vi "PatManage.vi"() -> ()   [LabVIEW 2012]
panel:
  in  "print":bool
  out "簇":T1
  in  "delete":bool
  in  "add":bool
  in  "ShowAll":bool
  in  "find":u16(ring) items=["请选择查询方式", "编号查询", "姓名查询", "性别查询", "年龄查询", "病区/床号查询", "治疗模式查询", "治疗次数查询", "治疗时长查询", "治疗日期查询"]
  out "查找结果":string
  in  "病历显示":string[][](table)
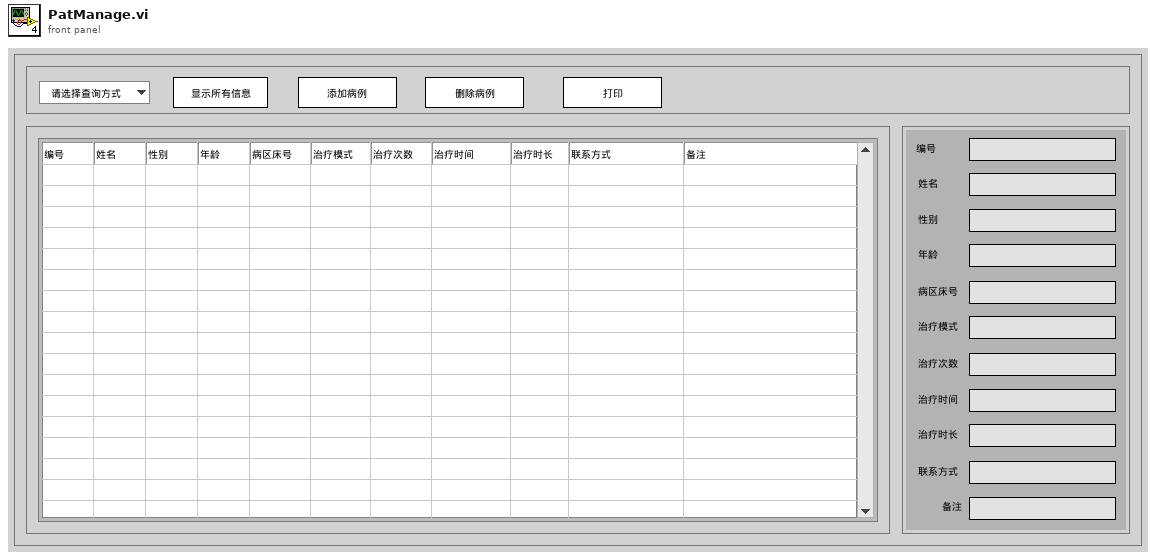
[diagram p1: front panel]
types:
  T1 = cluster{"编号":string, "姓名":string, "性别":string, "年龄":string, "病区床号":string, "治疗模式":string, "治疗次数":string, "治疗时间":string, "治疗时长":string, "联系方式":string, "备注":string}
  T2 = typedef "LVRowAndColumnTypeDef.ctl" = cluster{"Row":i32, "Column":i32}
  T3 = cluster{string, string, string, string, string, string, string, string, string, string, string}
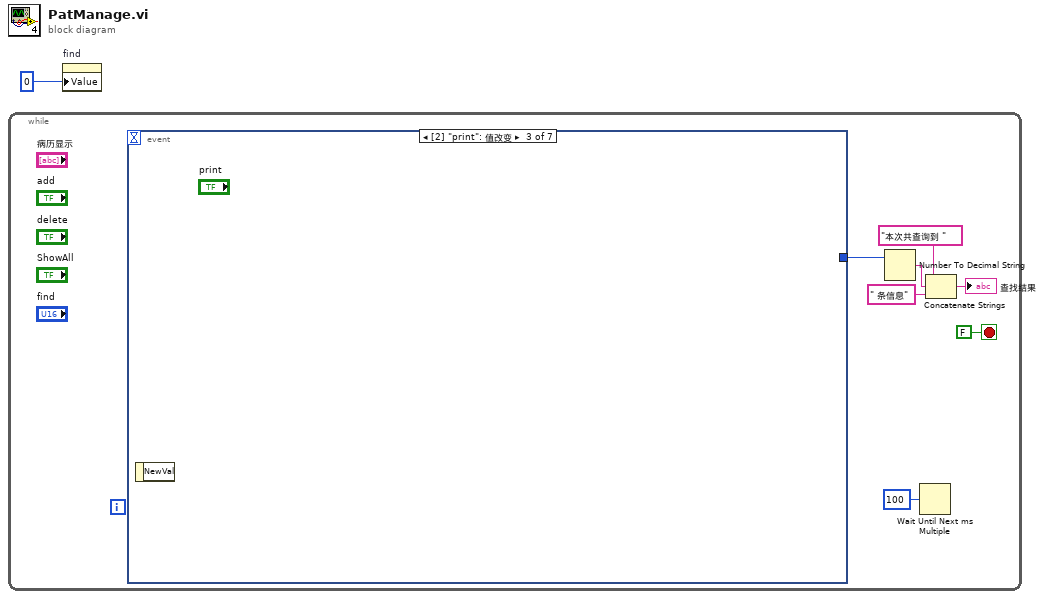
[diagram p0: block diagram]
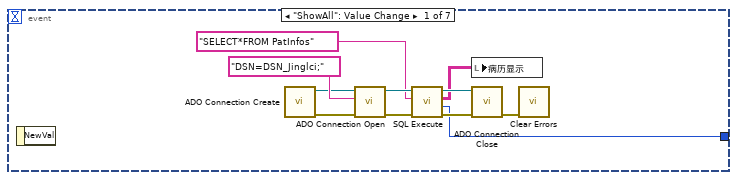
[diagram p2: hidden frame]
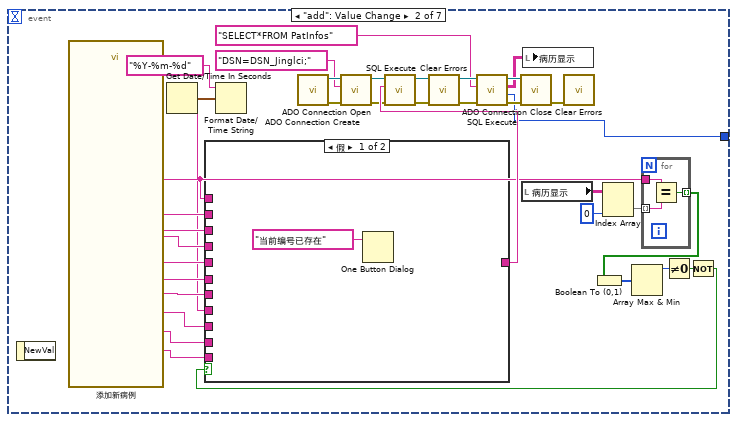
[diagram p3: hidden frame]
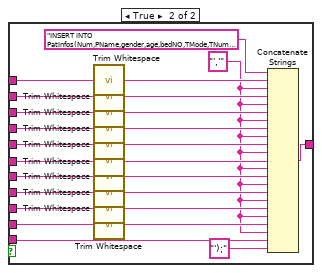
[diagram p4: hidden frame]
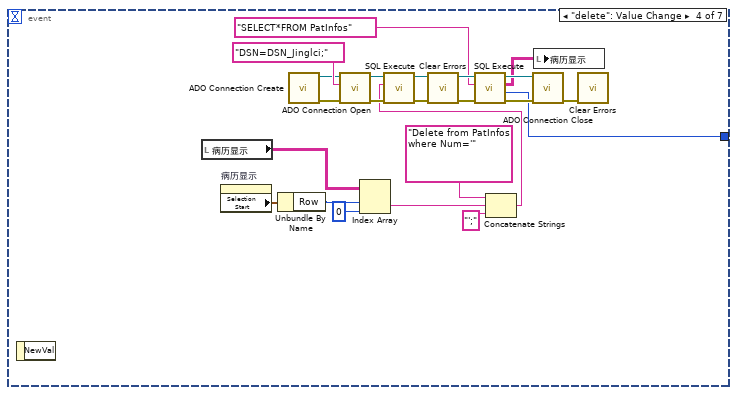
[diagram p5: hidden frame]
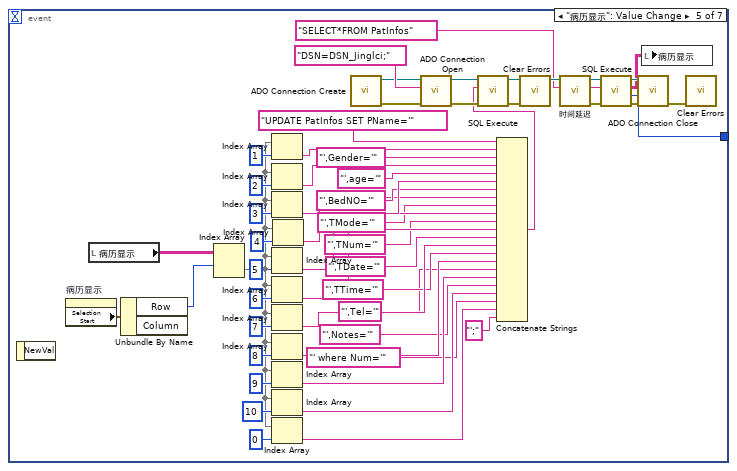
[diagram p6: hidden frame]
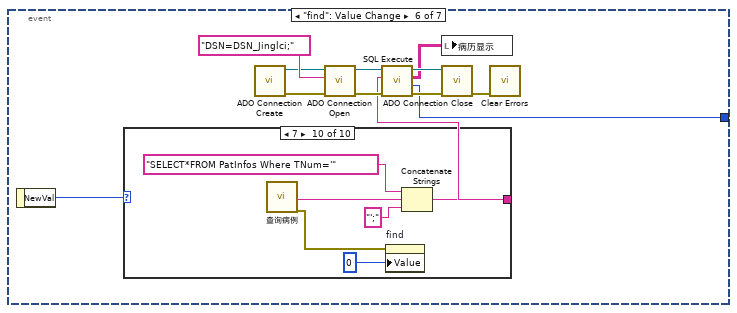
[diagram p7: hidden frame]
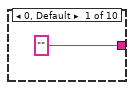
[diagram p8: hidden frame]
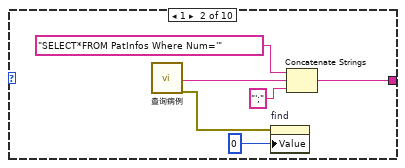
[diagram p9: hidden frame]
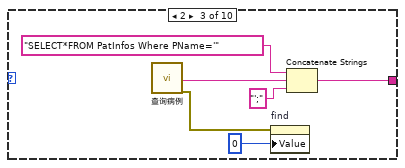
[diagram p10: hidden frame]
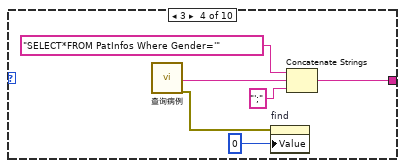
[diagram p11: hidden frame]
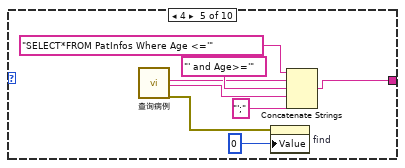
[diagram p12: hidden frame]
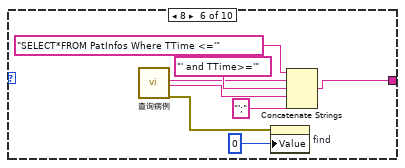
[diagram p13: hidden frame]
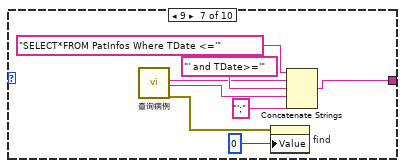
[diagram p14: hidden frame]
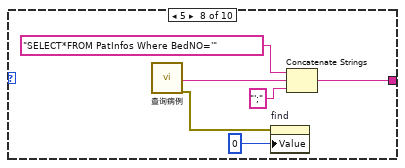
[diagram p15: hidden frame]
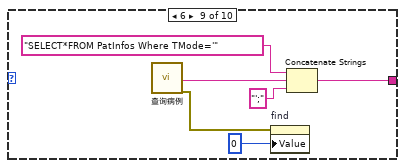
[diagram p16: hidden frame]
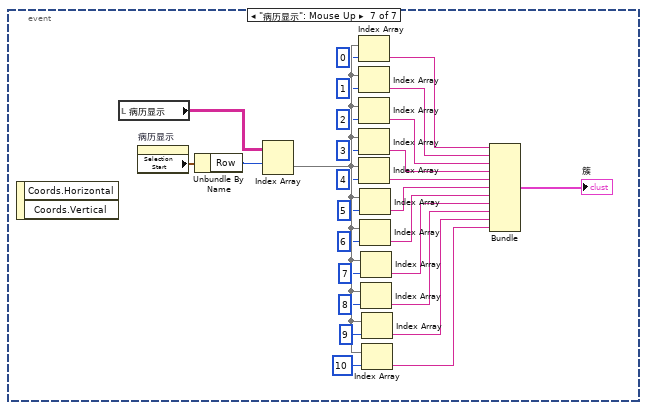
[diagram p17: hidden frame]
diagram:
  n1 = while {
    stop <- FALSE stop-if-true
    n2 = event shown="[2] \"print\": 值改变" {
      selector: _ -> [_ _ _ _ _ _ _]
      dyn-events: _ -> [_ _ _ _ _ _ _]
      timeout: _ -> [_ _ _ _ _ _ _]
      tunnel: [w9 w37 _ w88 w148 w160 _] -> w2
      event "ShowAll": Value Change {
        n3 = event-data() -> ()  [unwired: 1 in, 1 out]
        n4 = call "ADO Connection Create.vi"() -> ("error out"=w14:errorcluster, "ADODB._Connection Out"=w13:refnum<k7>)  [unwired: 10 in]
        n5 = call "ADO Connection Open.vi"("error in (no error)"=w14, "ConnectionString"="DSN=DSN_Jinglci;" ("Command Text"), "ADODB._Connection In"=w13) -> ("error out"=w19:errorcluster, "ADODB._Connection Out"=w18:refnum<k7>)  [unwired: 7 in]
        n6 = call "SQL Execute.vi"("error in (no error)"=w19, "Command Text"="SELECT*FROM PatInfos", "ADODB._Connection In"=w18) -> ("error out"=w15:errorcluster, "Rows Fetched"=w9:i32, "Data"=w10:string[][], "ADODB._Connection Out"=w17:refnum<k7>)  [unwired: 5 in]
        n7 = local write "病历显示"(w10) -> ()
        n8 = call "ADO Connection Close.vi"("error in (no error)"=w15, "ADODB._Connection In"=w17) -> ("error out"=w11:errorcluster)  [unwired: 8 in, 1 out]
        n9 = call <vilib>:"Clear Errors.vi"("error in (no error)"=w11) -> ()  [unwired: 6 in, 1 out]
      }
      event "add": Value Change {
        n10 = event-data() -> ()  [unwired: 1 in, 1 out]
        n11 = call "添加新病例"() -> ("备注"=w25:string, "联系方式"=w26:string, "治疗时长"=w22:string, "治疗次数"=w50:string, "治疗模式"=w51:string, "病区/床号"=w52:string, "年龄"=w53:string, "性别"=w54:string, "姓名"=w55:string, "编号"=w32:string)  [unwired: 8 in, 2 out]
        n12 = Get Date/Time In Seconds() -> (seconds since 1Jan1904=w24:timestamp)
        n13 = Format Date/Time String(time format string (%c)="%Y-%m-%d" ("时间格式字符串(%c)"), seconds (now)=w24) -> (date/time string=w21:string)  [unwired: 1 in]
        n14 = call "ADO Connection Create.vi"() -> ("error out"=w45:errorcluster, "ADODB._Connection Out"=w49:refnum<k7>)  [unwired: 10 in]
        n15 = call "ADO Connection Open.vi"("error in (no error)"=w45, "ConnectionString"="DSN=DSN_Jinglci;" ("Command Text"), "ADODB._Connection In"=w49) -> ("error out"=w44:errorcluster, "ADODB._Connection Out"=w47:refnum<k7>)  [unwired: 7 in]
        n16 = local read "病历显示"() -> (w34:string[][])
        n17 = Index Array(array=w34, index (col)=0 ("禁用的索引 (列)")) -> (element=w31:string[])  [unwired: 1 in]
        n18 = for {
          tunnel: w32 -> [w58]
          tunnel: w31 -> [w57] mode=indexing
          tunnel: [w56] -> w28 mode=indexing
          n19 = Equal?(x=w58, y=w57) -> (x = y?=w56:bool)
        }
        n20 = Boolean To (0,1)(Boolean=w28) -> (0, 1=w29:i16[])
        n21 = Array Max & Min(array=w29) -> (max value=w30:i16)  [unwired: 3 out]
        n22 = Not Equal To 0?(x=w30) -> (x != 0?=w27:bool)
        n23 = Not(x=w27) -> (.not. x?=w20:bool)
        n24 = case shown="假" w20 {
          tunnel: w32 -> [_ w84]
          tunnel: w55 -> [_ w83]
          tunnel: w54 -> [_ w82]
          tunnel: w53 -> [_ w81]
          tunnel: w52 -> [_ w80]
          tunnel: w51 -> [_ w79]
          tunnel: w50 -> [_ w78]
          tunnel: w21 -> [_ w77]
          tunnel: [_ w76] -> w46
          tunnel: w26 -> [_ w66]
          tunnel: w25 -> [_ w63]
          tunnel: w22 -> [_ w61]
          frame False {
            n25 = One Button Dialog(message="当前编号已存在" ("消息")) -> ()  [unwired: 1 in, 1 out]
          }
          frame True {
            w64 = "','"
            n26 = call <vilib>:"Trim Whitespace.vi"("string"=w84) -> ("trimmed string"=w75:string)  [unwired: 1 in]
            n27 = call <vilib>:"Trim Whitespace.vi"("string"=w83) -> ("trimmed string"=w74:string)  [unwired: 1 in]
            n28 = call <vilib>:"Trim Whitespace.vi"("string"=w82) -> ("trimmed string"=w73:string)  [unwired: 1 in]
            n29 = call <vilib>:"Trim Whitespace.vi"("string"=w81) -> ("trimmed string"=w72:string)  [unwired: 1 in]
            n30 = call <vilib>:"Trim Whitespace.vi"("string"=w80) -> ("trimmed string"=w71:string)  [unwired: 1 in]
            n31 = call <vilib>:"Trim Whitespace.vi"("string"=w79) -> ("trimmed string"=w70:string)  [unwired: 1 in]
            n32 = call <vilib>:"Trim Whitespace.vi"("string"=w78) -> ("trimmed string"=w69:string)  [unwired: 1 in]
            n33 = call <vilib>:"Trim Whitespace.vi"("string"=w77) -> ("trimmed string"=w68:string)  [unwired: 1 in]
            n34 = call <vilib>:"Trim Whitespace.vi"("string"=w61) -> ("trimmed string"=w67:string)  [unwired: 1 in]
            n35 = call <vilib>:"Trim Whitespace.vi"("string"=w66) -> ("trimmed string"=w65:string)  [unwired: 1 in]
            n36 = Concatenate Strings("INSERT INTO PatInfos(Num,PName,gender,age,bedNO,TMode,TNum,TDate,TTime,Tel,notes)VALUES('" ("Command Text"), w75, w64, w74, w64, w73, w64, w72, w64, w71, w64, w70, w64, w69, w64, w68, w64, w67, w64, w65, w64, w63, "');") -> (w76:string)
          }
        }
        n37 = call "SQL Execute.vi"("error in (no error)"=w44, "Command Text"=w46, "ADODB._Connection In"=w47) -> ("error out"=w42:errorcluster, "ADODB._Connection Out"=w41:refnum<k7>)  [unwired: 5 in, 2 out]
        n38 = call <vilib>:"Clear Errors.vi"("error in (no error)"=w42) -> ("error out"=w35:errorcluster)  [unwired: 6 in]
        n39 = call "SQL Execute.vi"("error in (no error)"=w35, "Command Text"="SELECT*FROM PatInfos", "ADODB._Connection In"=w41) -> ("error out"=w39:errorcluster, "Rows Fetched"=w37:i32, "Data"=w38:string[][], "ADODB._Connection Out"=w40:refnum<k7>)  [unwired: 5 in]
        n40 = call "ADO Connection Close.vi"("error in (no error)"=w39, "ADODB._Connection In"=w40) -> ("error out"=w43:errorcluster)  [unwired: 8 in, 1 out]
        n41 = local write "病历显示"(w38) -> ()
        n42 = call <vilib>:"Clear Errors.vi"("error in (no error)"=w43) -> ()  [unwired: 6 in, 1 out]
      }
      event "print": Value Change {
        n43 = event-data() -> ()  [unwired: 1 in, 1 out]
      }
      event "delete": Value Change {
        n44 = event-data() -> ()  [unwired: 1 in, 1 out]
        n45 = local read "病历显示"() -> (w103:string[][])
        n46 = property on="病历显示" class="Tbl (严格)"() -> ("Selection Start"=w106:T2)  [unwired: 2 in, 2 out]
        n47 = Unbundle By Name(w106) -> ("Row"=w104:i32)
        n48 = call "ADO Connection Create.vi"() -> ("error out"=w96:errorcluster, "ADODB._Connection Out"=w97:refnum<k7>)  [unwired: 10 in]
        n49 = call "ADO Connection Open.vi"("error in (no error)"=w96, "ConnectionString"="DSN=DSN_Jinglci;" ("Command Text"), "ADODB._Connection In"=w97) -> ("error out"=w95:errorcluster, "ADODB._Connection Out"=w99:refnum<k7>)  [unwired: 7 in]
        n50 = Index Array(array=w103, index (row)=w104, index (col)=0 ("disabled index (col)")) -> (element=w102:string)
        n51 = Concatenate Strings("Delete from PatInfos where Num='" ("SQL Text"), w102, "';" ("string")) -> (w93:string)
        n52 = call "SQL Execute.vi"("error in (no error)"=w95, "Command Text"=w93, "ADODB._Connection In"=w99) -> ("error out"=w86:errorcluster, "ADODB._Connection Out"=w92:refnum<k7>)  [unwired: 5 in, 2 out]
        n53 = call <vilib>:"Clear Errors.vi"("error in (no error)"=w86) -> ("error out"=w85:errorcluster)  [unwired: 6 in]
        n54 = call "SQL Execute.vi"("error in (no error)"=w85, "Command Text"="SELECT*FROM PatInfos", "ADODB._Connection In"=w92) -> ("error out"=w90:errorcluster, "Rows Fetched"=w88:i32, "Data"=w89:string[][], "ADODB._Connection Out"=w91:refnum<k7>)  [unwired: 5 in]
        n55 = call "ADO Connection Close.vi"("error in (no error)"=w90, "ADODB._Connection In"=w91) -> ("error out"=w94:errorcluster)  [unwired: 8 in, 1 out]
        n56 = local write "病历显示"(w89) -> ()
        n57 = call <vilib>:"Clear Errors.vi"("error in (no error)"=w94) -> ()  [unwired: 6 in, 1 out]
      }
      event "病历显示": Value Change {
        n58 = event-data() -> ()  [unwired: 1 in, 1 out]
        n59 = property on="病历显示" class="Tbl (严格)"() -> ("Selection Start"=w147:T2)  [unwired: 2 in, 2 out]
        n60 = local read "病历显示"() -> (w146:string[][])
        n61 = Unbundle By Name(w147) -> ("Row"=w145:i32)  [unwired: 1 out]
        n62 = Index Array(array=w146, index (row)=w145) -> (element=w112:string[])  [unwired: 1 in]
        n63 = Index Array(array=w112, index=1 ("索引")) -> (element=w126:string)
        n64 = Index Array(array=w112, index=2 ("索引")) -> (element=w140:string)
        n65 = Index Array(array=w112, index=3 ("索引")) -> (element=w137:string)
        n66 = Index Array(array=w112, index=5 ("索引")) -> (element=w132:string)
        n67 = Index Array(array=w112, index=6 ("索引")) -> (element=w130:string)
        n68 = Index Array(array=w112, index=7 ("索引")) -> (element=w124:string)
        n69 = Index Array(array=w112, index=8 ("索引")) -> (element=w121:string)
        n70 = Index Array(array=w112, index=9 ("索引")) -> (element=w119:string)
        n71 = Index Array(array=w112, index=10 ("索引")) -> (element=w113:string)
        n72 = Index Array(array=w112, index=0 ("索引")) -> (element=w111:string)
        n73 = Index Array(array=w112, index=4 ("索引")) -> (element=w134:string)
        n74 = call "ADO Connection Create.vi"() -> ("error out"=w156:errorcluster, "ADODB._Connection Out"=w155:refnum<k7>)  [unwired: 10 in]
        n75 = call "ADO Connection Open.vi"("error in (no error)"=w156, "ConnectionString"="DSN=DSN_Jinglci;" ("Command Text"), "ADODB._Connection In"=w155) -> ("error out"=w159:errorcluster, "ADODB._Connection Out"=w158:refnum<k7>)  [unwired: 7 in]
        n76 = Concatenate Strings("UPDATE PatInfos SET PName='" ("Command Text"), w126, "',Gender='" ("字符串"), w140, "',age='" ("字符串"), w137, "',BedNO='" ("字符串"), w134, "',TMode='" ("字符串"), w132, "',TNum='" ("字符串"), w130, "',TDate='" ("字符串"), w124, "',TTime='" ("字符串"), w121, "',Tel='" ("字符串"), w119, "',Notes='" ("字符串"), w113, "' where Num='" ("字符串"), w111, "';" ("字符串")) -> (w118:string)
        n77 = call "SQL Execute.vi"("error in (no error)"=w159, "Command Text"=w118, "ADODB._Connection In"=w158) -> ("error out"=w117:errorcluster, "ADODB._Connection Out"=w153:refnum<k7>)  [unwired: 5 in, 2 out]
        n78 = call <vilib>:"Clear Errors.vi"("error in (no error)"=w117) -> ()  [unwired: 6 in, 1 out]
        n79 = call "时间延迟"() -> ("error out"=w116:errorcluster)  [unwired: 11 in]
        n80 = call "SQL Execute.vi"("error in (no error)"=w116, "Command Text"="SELECT*FROM PatInfos", "ADODB._Connection In"=w153) -> ("error out"=w151:errorcluster, "Rows Fetched"=w148:i32, "Data"=w149:string[][], "ADODB._Connection Out"=w152:refnum<k7>)  [unwired: 5 in]
        n81 = call "ADO Connection Close.vi"("error in (no error)"=w151, "ADODB._Connection In"=w152) -> ("error out"=w154:errorcluster)  [unwired: 8 in, 1 out]
        n82 = local write "病历显示"(w149) -> ()
        n83 = call <vilib>:"Clear Errors.vi"("error in (no error)"=w154) -> ()  [unwired: 6 in, 1 out]
      }
      event "find": Value Change {
        n84 = event-data() -> ("NewVal"=w171:u16)  [unwired: 1 in]
        n85 = case shown="7" w171 {
          tunnel: ["" w175 w182 w188 w191 w199 w207 w218 w224 w230] -> w163
          frame 0, Default {
          }
          frame 1 {
            n86 = call "查询病例"() -> ("病例编号"=w177:string, "error out"=w173:errorcluster)  [unwired: 17 in, 1 out]
            n87 = property on="find" class="Ring (严格)"(error in=w173, "Value"=0) -> ()  [unwired: 1 in, 2 out]
            n88 = Concatenate Strings("SELECT*FROM PatInfos Where Num='" ("Command Text"), w177, "';") -> (w175:string)
          }
          frame 2 {
            n89 = call "查询病例"() -> ("病例姓名"=w181:string, "error out"=w180:errorcluster)  [unwired: 17 in, 1 out]
            n90 = property on="find" class="Ring (严格)"(error in=w180, "Value"=0) -> ()  [unwired: 1 in, 2 out]
            n91 = Concatenate Strings("SELECT*FROM PatInfos Where PName='" ("Command Text"), w181, "';") -> (w182:string)
          }
          frame 3 {
            n92 = call "查询病例"() -> ("病例性别"=w187:string, "error out"=w186:errorcluster)  [unwired: 17 in, 1 out]
            n93 = property on="find" class="Ring (严格)"(error in=w186, "Value"=0) -> ()  [unwired: 1 in, 2 out]
            n94 = Concatenate Strings("SELECT*FROM PatInfos Where Gender='" ("Command Text"), w187, "';") -> (w188:string)
          }
          frame 4 {
            n95 = call "查询病例"() -> ("病例年龄上限"=w195:string, "病例年龄下限"=w194:string, "error out"=w197:errorcluster)  [unwired: 16 in, 1 out]
            n96 = property on="find" class="Ring (严格)"(error in=w197, "Value"=0) -> ()  [unwired: 1 in, 2 out]
            n97 = Concatenate Strings("SELECT*FROM PatInfos Where Age <='" ("Command Text"), w195, "' and Age>='", w194, "';" ("字符串")) -> (w191:string)
          }
          frame 8 {
            n98 = call "查询病例"() -> ("治疗时长上限"=w203:string, "治疗时长下限"=w202:string, "error out"=w205:errorcluster)  [unwired: 16 in, 1 out]
            n99 = property on="find" class="Ring (严格)"(error in=w205, "Value"=0) -> ()  [unwired: 1 in, 2 out]
            n100 = Concatenate Strings("SELECT*FROM PatInfos Where TTime <='" ("Command Text"), w203, "' and TTime>='", w202, "';" ("字符串")) -> (w199:string)
          }
          frame 9 {
            n101 = call "查询病例"() -> ("截止日期"=w211:string, "起始日期"=w210:string, "error out"=w213:errorcluster)  [unwired: 16 in, 1 out]
            n102 = property on="find" class="Ring (严格)"(error in=w213, "Value"=0) -> ()  [unwired: 1 in, 2 out]
            n103 = Concatenate Strings("SELECT*FROM PatInfos Where TDate <='" ("Command Text"), w211, "' and TDate>='", w210, "';" ("字符串")) -> (w207:string)
          }
          frame 5 {
            n104 = call "查询病例"() -> ("病例所在病区、床号"=w217:string, "error out"=w216:errorcluster)  [unwired: 17 in, 1 out]
            n105 = property on="find" class="Ring (严格)"(error in=w216, "Value"=0) -> ()  [unwired: 1 in, 2 out]
            n106 = Concatenate Strings("SELECT*FROM PatInfos Where BedNO='" ("Command Text"), w217, "';") -> (w218:string)
          }
          frame 6 {
            n107 = call "查询病例"() -> ("治疗模式"=w223:string, "error out"=w222:errorcluster)  [unwired: 17 in, 1 out]
            n108 = property on="find" class="Ring (严格)"(error in=w222, "Value"=0) -> ()  [unwired: 1 in, 2 out]
            n109 = Concatenate Strings("SELECT*FROM PatInfos Where TMode='" ("Command Text"), w223, "';") -> (w224:string)
          }
          frame 7 {
            n110 = call "查询病例"() -> ("治疗次数"=w229:string, "error out"=w228:errorcluster)  [unwired: 17 in, 1 out]
            n111 = property on="find" class="Ring (严格)"(error in=w228, "Value"=0) -> ()  [unwired: 1 in, 2 out]
            n112 = Concatenate Strings("SELECT*FROM PatInfos Where TNum='" ("Command Text"), w229, "';") -> (w230:string)
          }
        }
        n113 = call "ADO Connection Create.vi"() -> ("error out"=w165:errorcluster, "ADODB._Connection Out"=w164:refnum<k7>)  [unwired: 10 in]
        n114 = call "ADO Connection Open.vi"("error in (no error)"=w165, "ConnectionString"="DSN=DSN_Jinglci;" ("Command Text"), "ADODB._Connection In"=w164) -> ("error out"=w170:errorcluster, "ADODB._Connection Out"=w169:refnum<k7>)  [unwired: 7 in]
        n115 = call "SQL Execute.vi"("error in (no error)"=w170, "Command Text"=w163, "ADODB._Connection In"=w169) -> ("error out"=w166:errorcluster, "Rows Fetched"=w160:i32, "Data"=w161:string[][], "ADODB._Connection Out"=w168:refnum<k7>)  [unwired: 5 in]
        n116 = local write "病历显示"(w161) -> ()
        n117 = call "ADO Connection Close.vi"("error in (no error)"=w166, "ADODB._Connection In"=w168) -> ("error out"=w162:errorcluster)  [unwired: 8 in, 1 out]
        n118 = call <vilib>:"Clear Errors.vi"("error in (no error)"=w162) -> ()  [unwired: 6 in, 1 out]
      }
      event "病历显示": Mouse Up {
        n119 = event-data() -> ()  [unwired: 1 in, 2 out]
        n120 = local read "病历显示"() -> (w257:string[][])
        n121 = property on="病历显示" class="Tbl (严格)"() -> ("Selection Start"=w259:T2)  [unwired: 2 in, 2 out]
        n122 = Unbundle By Name(w259) -> ("Row"=w258:i32)
        n123 = Index Array(array=w257, index (row)=w258) -> (element=w256:string[])  [unwired: 1 in]
        n124 = Index Array(array=w256, index=0 ("索引")) -> (element=w254:string)
        n125 = Index Array(array=w256, index=1 ("索引")) -> (element=w253:string)
        n126 = Index Array(array=w256, index=2 ("索引")) -> (element=w252:string)
        n127 = Index Array(array=w256, index=3 ("索引")) -> (element=w251:string)
        n128 = Index Array(array=w256, index=4 ("索引")) -> (element=w250:string)
        n129 = Index Array(array=w256, index=5 ("索引")) -> (element=w249:string)
        n130 = Index Array(array=w256, index=6 ("索引")) -> (element=w248:string)
        n131 = Index Array(array=w256, index=7 ("索引")) -> (element=w247:string)
        n132 = Index Array(array=w256, index=8 ("索引")) -> (element=w246:string)
        n133 = Index Array(array=w256, index=9 ("索引")) -> (element=w245:string)
        n134 = Index Array(array=w256, index=10 ("索引")) -> (element=w244:string)
        n135 = Bundle(w254, w253, w252, w251, w250, w249, w248, w247, w246, w245, w244) -> (→"簇":T3)  [unwired: 1 in]
      }
    }
    n136 = Number To Decimal String(number=w2) -> (decimal integer string=w4:string)  [unwired: 1 in]
    n137 = Wait Until Next ms Multiple(millisecond multiple=u32 100 ("毫秒倍数")) -> ()  [unwired: 1 out]
    n138 = Concatenate Strings("本次共查询到 ", w4, " 条信息") -> (→"查找结果":string)
  }
  n139 = property on="find" class="Ring (严格)"("Value"=0) -> ()  [unwired: 2 in, 2 out]
